vi "Construct.vi"(0 "Components":refnum<class "Component.lvclass">[](array[class]), 11 "error in (no error)":errorcluster) -> (4 "Build Analyzer":refnum<class "Build Analyzer.lvclass">, 15 "error out":errorcluster)   [LabVIEW 2017, in "CL_G3_VIComponentBuilder.lvlib" / "Build Analyzer.lvclass"]
doc: "Generates a hierarchy of components based on an array of \"Component Definition.ini\" files. The set of discovered components is the working set from which build order is determined."
uses:
  Build Analyzer.lvclass
  Components/Component.lvclass
  Exports/Exports/Export.lvclass
  Components/Component.lvclass/Component.ctl
  Build Analyzer.lvclass/Build Analyzer.ctl
  Exports/Exports/Export.lvclass/Export.ctl
  <userlib>/_Cirrus Logic/LabVIEW Container/Source/Container/Container.lvclass/Container.ctl
  Components/Accessors/Read Component Config File.vi
  Components/Accessors/Read Product Name.vi
  Components/Accessors/Read Unique Name.vi
  Accessors/Write Components.vi
  Accessors/Write Component Product Name -_ Unique Name.vi
  <userlib>/_Cirrus Logic/LabVIEW Container/Source/Container/Set N Attributes.vi
  Exports/Exports/Accessors/Read unique Name.vi
  Exports/Exports/Accessors/Read Product Name.vi
  Exports/Exports/Accessors/Read Export Build Specification.vi
  Exports/Exports/Accessors/Read Dependencies' Unique Names.vi
  Exports/Exports/Accessors/Read Owning Component's Product Name.vi
  Exports/Exports/Accessors/Read Owning Component's Unique Name.vi
  Accessors/Write Top Down Working Set.vi
  Accessors/Write Bubble Up Working Set.vi
  <userlib>/_Cirrus Logic/LabVIEW Container/Source/Container/SubVIs/SetAttribute_ByValue.vi
  <userlib>/_Cirrus Logic/LabVIEW Container/Source/Container/Get Child.vi
  <userlib>/_Cirrus Logic/LabVIEW Container/Source/Container/GetAttribute_Path.vi
  <userlib>/_Cirrus Logic/LabVIEW Container/Source/CIR/Interface Definition/Container Intermediate Representation.lvclass
  <userlib>/_Cirrus Logic/LabVIEW Container/Source/Container/Container.lvclass
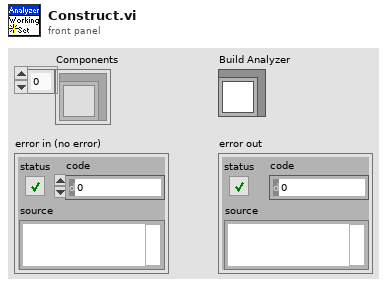
[diagram p1: front panel]
types:
  T1 = cluster{"Build Analyzer":refnum<class "Build Analyzer.lvclass">, "Components":refnum<class "Component.lvclass">[], "Exports":refnum<class "Export.lvclass">[]}
  T2 = enum16{"Overwrite Conflicts", "Error on Conflicts"}
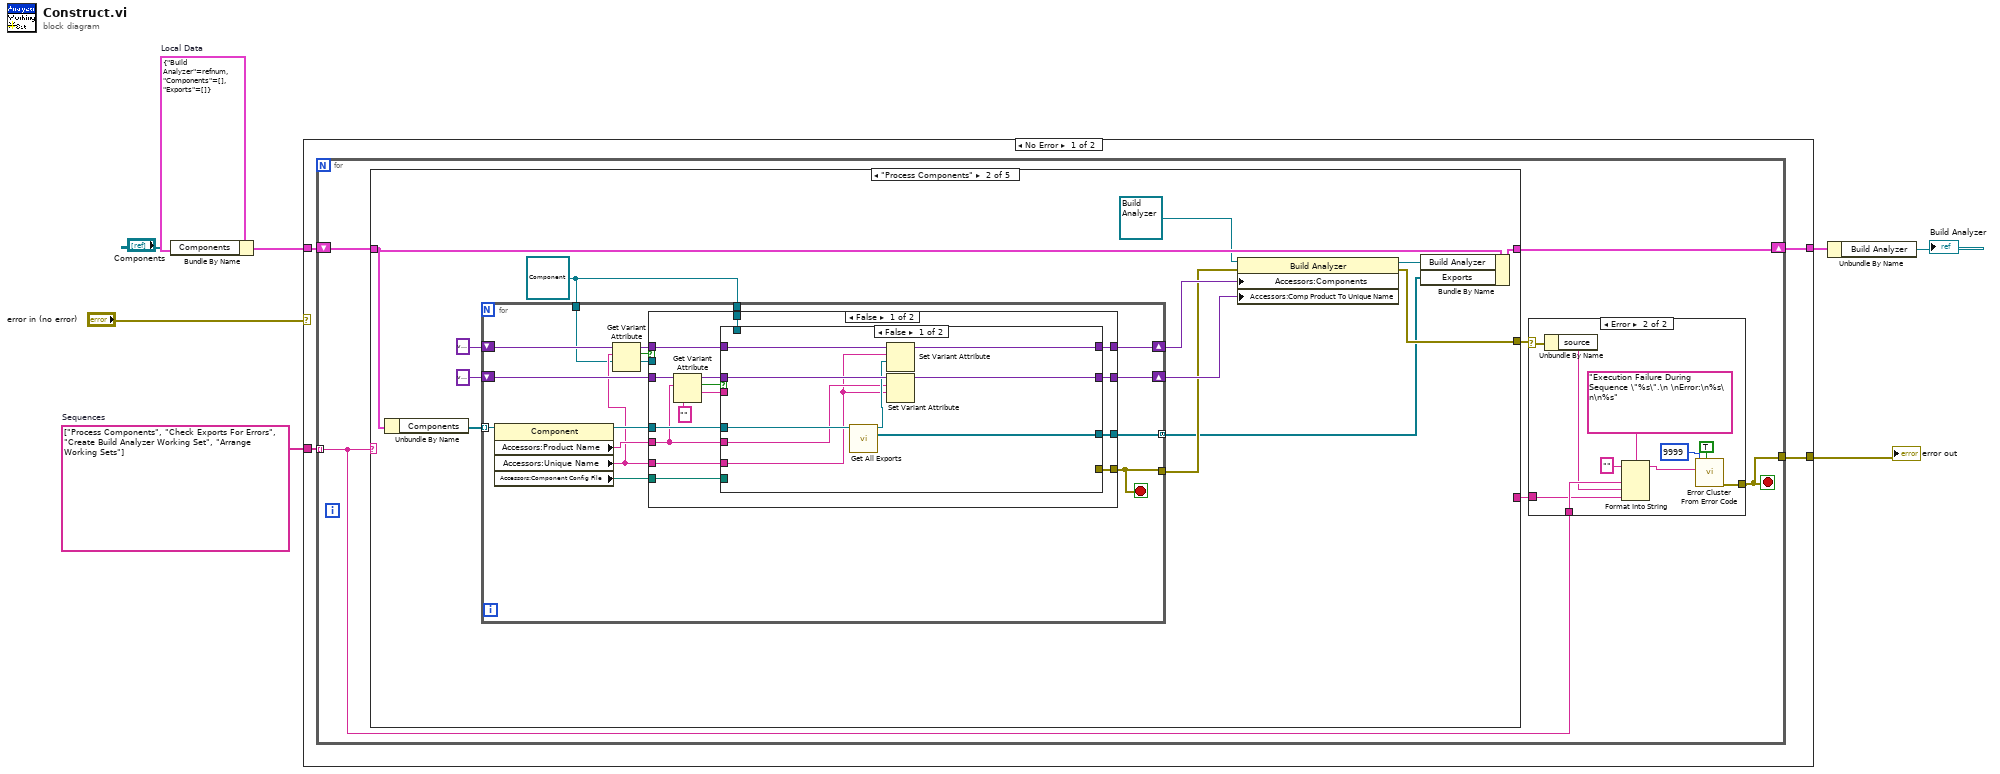
[diagram p0: block diagram]
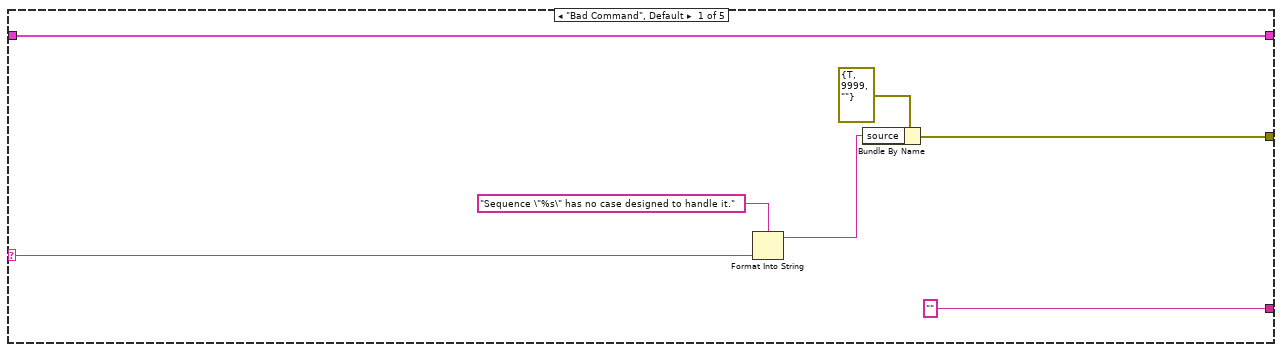
[diagram p3: hidden frame]
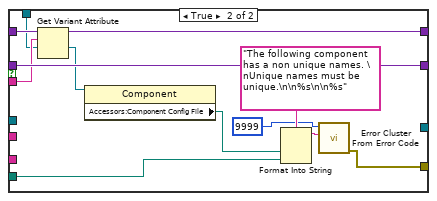
[diagram p4: hidden frame]
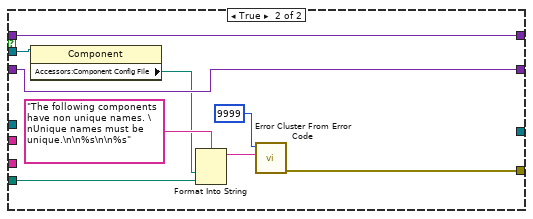
[diagram p5: hidden frame]
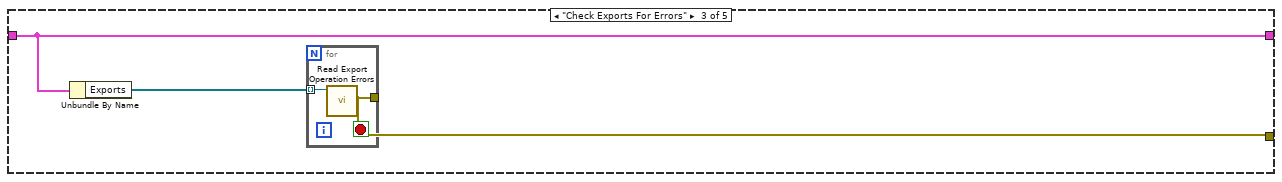
[diagram p6: hidden frame]
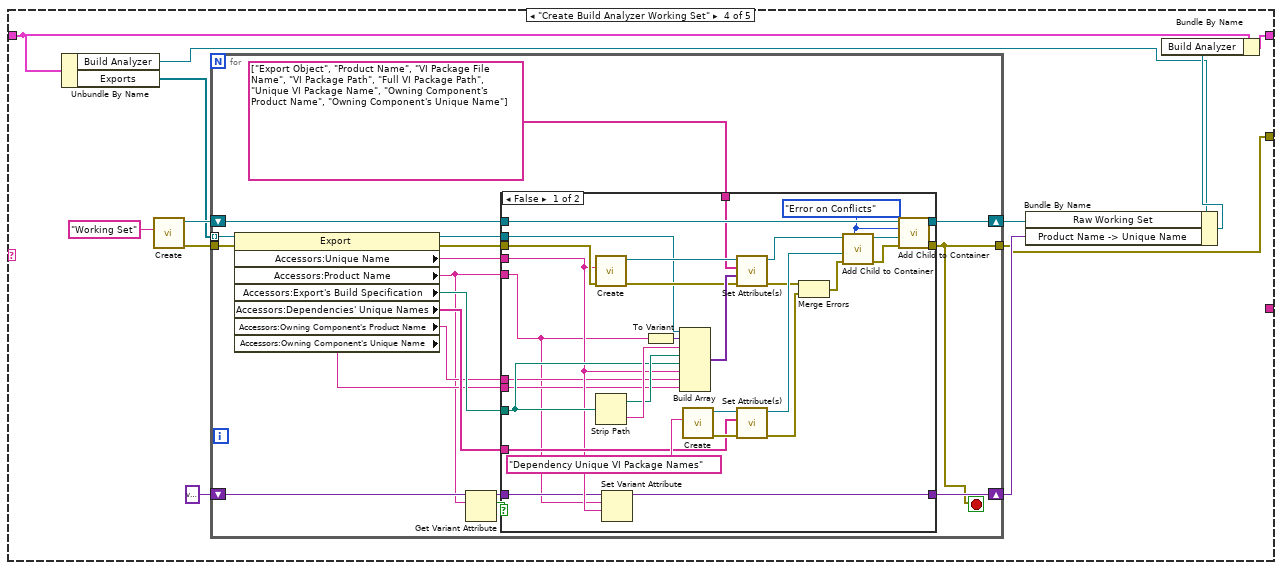
[diagram p7: hidden frame]
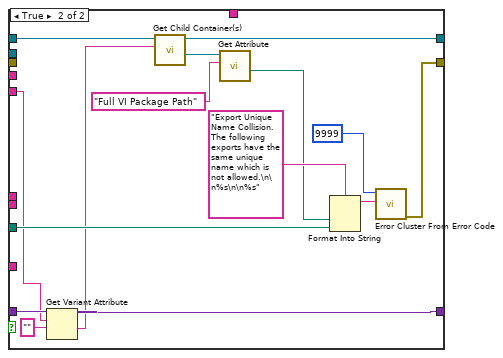
[diagram p8: hidden frame]
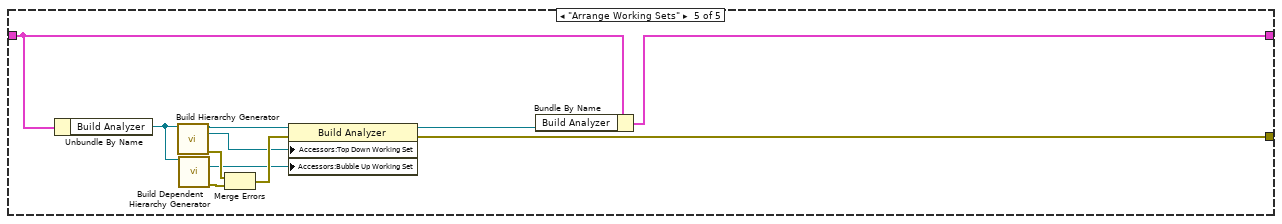
[diagram p9: hidden frame]
diagram:
  w5 = T1 {"Build Analyzer"=refnum, "Components"=[], "Exports"=[]}  # Local Data
  w7 = string[] ["Process Components", "Check Exports For Errors", "Create Build Analyzer Working Set", "Arrange Working Sets"]  # Sequences
  n1 = Bundle By Name(cluster=w5, "Components"="Components") -> (w8:T1)
  n2 = case shown="No Error" "error in (no error)" {
    selector: "error in (no error)" -> [_ w203]
    tunnel: w7 -> [w12 _]
    tunnel: w8 -> [w11 w204]
    tunnel: [w10 w204] -> w6
    tunnel: [w9 w203] -> w2
    frame No Error {
      n3 = for {
        tunnel: w12 -> [w15] mode=indexing
        shift-right: [w17] -> w10
        shift-left: w11 -> [w18]
        tunnel: [w13] -> w9
        stop <- w13 stop-if-true
        n4 = case shown="\"Process Components\"" w15 {
          selector: w15 -> [w31 _ _ _ _]
          tunnel: w18 -> [w36 w47 w113 w123 w202]
          tunnel: [w36 w44 w113 w122 w195] -> w17
          tunnel: [w33 w38 w112 w118 w193] -> w16
          tunnel: ["" ("Accessors:Name") _ _ _ _] -> w14
          frame "Bad Command", Default {
            n5 = Format Into String(format string="Sequence \"%s\" has no case designed to handle it.", w31) -> (resulting string=w30:string)  [unwired: 2 in, 1 out]
            n6 = Bundle By Name(cluster=errorcluster {"status"=TRUE, "code"=9999, "source"=""} ("error out"), "source"=w30) -> (w33:errorcluster)
          }
          frame "Process Components" {
            w43 = refnum<class "Component.lvclass"> refnum ("reference out")
            n7 = Unbundle By Name(w47) -> ("Components"=w46:refnum<class "Component.lvclass">[])
            n8 = for {
              tunnel: [w65] -> w37 mode=concatenating
              shift-right: [w64] -> w41
              shift-left: variant -> [w60]
              shift-right: [w63] -> w42
              shift-left: variant -> [w59]
              tunnel: w46 -> [w61] mode=indexing
              tunnel: [w54] -> w39
              tunnel: w43 -> [w51]
              tunnel: w43 -> [w50]
              stop <- w54 stop-if-true
              n9 = property class="Component"(reference=w61) -> (reference out=w62:refnum<class "Component.lvclass">, "Accessors:Product Name"=w53:string, "Accessors:Unique Name"=w52:string, "Accessors:Component Config File"=w55:path)  [unwired: 1 in, 1 out]
              n10 = Get Variant Attribute(Variant=w59, name=w52, default value (empty Variant)=w51) -> (duplicate Variant=w58:variant, found=w57:bool, value=w56:refnum<class "Component.lvclass">)  [unwired: 1 in, 1 out]
              n11 = case shown="False" w57 {
                tunnel: [w80 _] -> w65
                tunnel: [w79 w108] -> w64
                tunnel: [w78 w109] -> w63
                tunnel: w62 -> [w77 _]
                tunnel: w60 -> [w76 w108]
                tunnel: w58 -> [w70 w109]
                tunnel: w53 -> [w67 _]
                tunnel: w52 -> [w71 _]
                tunnel: w56 -> [_ w110]
                tunnel: w55 -> [w72 w105]
                tunnel: [w73 w103] -> w54
                tunnel: w50 -> [w66 _]
                frame False {
                  n12 = Get Variant Attribute(Variant=w76, name=w67, default value (empty Variant)="") -> (duplicate Variant=w75:variant, found=w74:bool, value=w68:string)  [unwired: 1 in, 1 out]
                  n13 = case shown="False" w74 {
                    tunnel: [w89 _] -> w80
                    tunnel: [w88 w101] -> w79
                    tunnel: [w87 w94] -> w78
                    tunnel: w77 -> [w86 _]
                    tunnel: w75 -> [w85 w101]
                    tunnel: w70 -> [w83 w96]
                    tunnel: w67 -> [w82 _]
                    tunnel: w71 -> [w81 _]
                    tunnel: [_ w98] -> w73
                    tunnel: w72 -> [_ w97]
                    tunnel: w68 -> [_ w95]
                    tunnel: w66 -> [_ w90]
                    frame False {
                      n14 = call "Get All Exports.vi"("Component in"=w86) -> ("Component out"=w84:refnum<class "Component.lvclass">, "Exports"=w89:refnum<class "Export.lvclass">[])  [unwired: 13 in]
                      n15 = Set Variant Attribute(Variant=w83, name=w81, value=w84) -> (Variant out=w87:variant)  [unwired: 1 in, 2 out]
                      n16 = Set Variant Attribute(Variant=w85, name=w82, value=w81) -> (Variant out=w88:variant)  [unwired: 1 in, 2 out]
                    }
                    frame True {
                      n17 = Get Variant Attribute(Variant=w96, name=w95, default value (empty Variant)=w90) -> (duplicate Variant=w94:variant, value=w93:refnum<class "Component.lvclass">)  [unwired: 1 in, 2 out]
                      n18 = property class="Component"(reference=w93) -> ("Accessors:Component Config File"=w92:path)  [unwired: 1 in, 2 out]
                      n19 = Format Into String(format string="The following component has a non unique names. \nUnique names must be unique.\n\n%s\n\n%s", w92, w97) -> (resulting string=w100:string)  [unwired: 2 in, 1 out]
                      n20 = call <vilib>:"Error Cluster From Error Code.vi"("error message (\"\")"=w100, "error code (0)"=9999) -> ("error out"=w98:errorcluster)  [unwired: 7 in]
                    }
                  }
                }
                frame True {
                  n21 = property class="Component"(reference=w110) -> ("Accessors:Component Config File"=w106:path)  [unwired: 1 in, 2 out]
                  n22 = Format Into String(format string="The following components have non unique names. \nUnique names must be unique.\n\n%s\n\n%s", w106, w105) -> (resulting string=w104:string)  [unwired: 2 in, 1 out]
                  n23 = call <vilib>:"Error Cluster From Error Code.vi"("error message (\"\")"=w104, "error code (0)"=9999) -> ("error out"=w103:errorcluster)  [unwired: 7 in]
                }
              }
            }
            n24 = property class="Build Analyzer"(reference=refnum<class "Build Analyzer.lvclass"> refnum ("Build Analyzer.lvclass"), error in=w39, "Accessors:Components"=w42, "Accessors:Comp Product To Unique Name"=w41) -> (reference out=w40:refnum<class "Build Analyzer.lvclass">, error out=w38:errorcluster)
            n25 = Bundle By Name(cluster=w47, "Build Analyzer"=w40, "Exports"=w37) -> (w44:T1)
          }
          frame "Check Exports For Errors" {
            n26 = Unbundle By Name(w113) -> ("Exports"=w111:refnum<class "Export.lvclass">[])
            n27 = for {
              tunnel: w111 -> [w115] mode=indexing
              tunnel: [w114] -> w112
              stop <- w114 stop-if-true
              n28 = call "Read Export Operation Errors.vi"("Export in"=w115) -> ("Export Operation Errors"=w114:errorcluster)  [unwired: 8 in, 2 out]
            }
          }
          frame "Create Build Analyzer Working Set" {
            n29 = Unbundle By Name(w123) -> ("Build Analyzer"=w117:refnum<class "Build Analyzer.lvclass">, "Exports"=w116:refnum<class "Export.lvclass">[])
            n30 = call <userlib>:"Create.vi"("Container Name"="Working Set") -> ("error out"=w125:errorcluster, "Container"=w127:refnum<data-value>)  [unwired: 9 in]
            n31 = for {
              shift-right: [w143] -> w120
              shift-left: w127 -> [w145]
              tunnel: w116 -> [w137] mode=indexing
              shift-right: [w138] -> w119
              shift-left: variant -> [w133]
              tunnel: w125 -> [w136]
              tunnel: [w131] -> w118
              stop <- w131 stop-if-true
              n32 = property class="Export"(reference=w137, error in=w136) -> (reference out=w140:refnum<class "Export.lvclass">, error out=w141:errorcluster, "Accessors:Unique Name"=w129:string, "Accessors:Product Name"=w128:string, "Accessors:Export's Build Specification"=w142:path, "Accessors:Dependencies' Unique Names"=w139:string[], "Accessors:Owning Component's Product Name"=w135:string, "Accessors:Owning Component's Unique Name"=w134:string)
              n33 = Get Variant Attribute(Variant=w133, name=w128) -> (duplicate Variant=w132:variant, found=w130:bool)  [unwired: 2 in, 2 out]
              n34 = case shown="False" w130 {
                tunnel: w145 -> [w176 w184]
                tunnel: string[] ["Export Object", "Product Name", "VI Package File Name", "VI Package Path", "Full VI Package Path", "Unique VI Package Name", "Owning Component's Product Name", "Owning Component's Unique Name"] ("Attribute Names") -> [w174 _]
                tunnel: [w169 w182] -> w143
                tunnel: w142 -> [w163 w189]
                tunnel: w141 -> [w162 _]
                tunnel: w140 -> [w155 _]
                tunnel: w139 -> [w154 _]
                tunnel: [w153 w177] -> w138
                tunnel: w129 -> [w152 _]
                tunnel: w135 -> [w151 _]
                tunnel: w134 -> [w150 _]
                tunnel: w132 -> [w149 w181]
                tunnel: w128 -> [w148 w180]
                tunnel: [w147 w186] -> w131
                frame False {
                  w146 = T2."Error on Conflicts" ("Overwrite behavior")
                  n35 = call <userlib>:"Create.vi"("error in (no error)"=w162, "Container Name"=w152) -> ("error out"=w161:errorcluster, "Container"=w175:refnum<data-value>)  [unwired: 8 in]
                  n36 = Strip Path(path=w163) -> (stripped path=w172:path, name=w173:string)
                  n37 = Set Variant Attribute(Variant=w149, name=w148, value=w152) -> (Variant out=w153:variant)  [unwired: 1 in, 2 out]
                  n38 = To Variant(anything=w148) -> (Variant=w170:variant)
                  n39 = Build Array(w155, w170, w173, w172, w163, w152, w151, w150) -> (w171:variant[])
                  n40 = call <userlib>:"Create.vi"("Container Name"="Dependency Unique VI Package Names") -> ("error out"=w160:errorcluster, "Container"=w165:refnum<data-value>)  [unwired: 9 in]
                  n41 = call-poly <userlib>:"Set Attribute(s).vi"("error in"=w161, "Attribute Values"=w171, "Attribute Names"=w174, "Container"=w175) -> ("error out"=w159:errorcluster, "Container out"=w167:refnum<data-value>)  [unwired: 5 in, 1 out]
                  n42 = call-poly <userlib>:"Set Attribute(s).vi"("error in"=w160, "Attribute Names"=w154, "Container"=w165) -> ("error out"=w158:errorcluster, "Container out"=w164:refnum<data-value>)  [unwired: 6 in, 1 out]
                  n43 = Merge Errors(w159, w158) -> (w157:errorcluster)
                  n44 = call <userlib>:"Add Child to Container.vi"("Overwrite behavior"=w146, "error in (no error)"=w157, "Child Container"=w164, "Container"=w167) -> ("error out"=w156:errorcluster, "dup Container"=w166:refnum<data-value>)  [unwired: 5 in, 1 out]
                  n45 = call <userlib>:"Add Child to Container.vi"("Overwrite behavior"=w146, "error in (no error)"=w156, "Child Container"=w166, "Container"=w176) -> ("error out"=w147:errorcluster, "dup Container"=w169:refnum<data-value>)  [unwired: 5 in, 1 out]
                }
                frame True {
                  n46 = Get Variant Attribute(Variant=w181, name=w180, default value (empty Variant)="") -> (duplicate Variant=w177:variant, value=w178:string)  [unwired: 1 in, 2 out]
                  n47 = call-poly <userlib>:"Get Child Container(s).vi"("Container Name"=w178, "Container"=w184) -> ("Child Container"=w183:refnum<data-value>, "dup Container"=w182:refnum<data-value>)  [unwired: 6 in, 2 out]
                  n48 = call-poly <userlib>:"Get Attribute.vi"("Attribute Name"="Full VI Package Path", "Container Reference"=w183) -> ("Path"=w188:path)  [unwired: 6 in, 3 out]
                  n49 = Format Into String(format string="Export Unique Name Collision. The following exports have the same unique name which is not allowed.\n\n%s\n\n%s", w188, w189) -> (resulting string=w187:string)  [unwired: 2 in, 1 out]
                  n50 = call <vilib>:"Error Cluster From Error Code.vi"("error message (\"\")"=w187, "error code (0)"=9999) -> ("error out"=w186:errorcluster)  [unwired: 7 in]
                }
              }
            }
            n51 = Bundle By Name(cluster=w117, "Raw Working Set"=w120, "Product Name -> Unique Name"=w119) -> (w121:refnum<class "Build Analyzer.lvclass">)
            n52 = Bundle By Name(cluster=w123, "Build Analyzer"=w121) -> (w122:T1)
          }
          frame "Arrange Working Sets" {
            n53 = Unbundle By Name(w202) -> ("Build Analyzer"=w196:refnum<class "Build Analyzer.lvclass">)
            n54 = call "Build Hierarchy Generator.vi"("Build Analyzer in"=w196) -> ("dup Build Analyzer"=w192:refnum<class "Build Analyzer.lvclass">, "Top Down Working Set"=w197:refnum<data-value>, "error out"=w201:errorcluster)  [unwired: 12 in]
            n55 = call "Build Dependent Hierarchy Generator.vi"("Build Analyzer in"=w196) -> ("Bubbe Up Working Set"=w198:refnum<data-value>, "error out"=w200:errorcluster)  [unwired: 12 in, 1 out]
            n56 = Merge Errors(w201, w200) -> (w199:errorcluster)
            n57 = property class="Build Analyzer"(reference=w192, error in=w199, "Accessors:Top Down Working Set"=w197, "Accessors:Bubble Up Working Set"=w198) -> (reference out=w194:refnum<class "Build Analyzer.lvclass">, error out=w193:errorcluster)
            n58 = Bundle By Name(cluster=w202, "Build Analyzer"=w194) -> (w195:T1)
          }
        }
        n59 = case shown="Error" w16 {
          selector: w16 -> [w19 w22]
          tunnel: [w19 w27] -> w13
          tunnel: w15 -> [_ w25]
          tunnel: w14 -> [_ w20]
          frame No Error {
          }
          frame Error {
            n60 = Unbundle By Name(w22) -> ("source"=w21:string)
            n61 = Format Into String(format string="Execution Failure During Sequence \"%s\".\n \nError:\n%s\n\n%s" ("error message (\"\")"), initial string="", w25, w21, w20) -> (resulting string=w26:string)  [unwired: 1 in, 1 out]
            n62 = call <vilib>:"Error Cluster From Error Code.vi"("show call chain? (False)"=TRUE, "error message (\"\")"=w26, "error code (0)"=9999) -> ("error out"=w27:errorcluster)  [unwired: 6 in]
          }
        }
      }
    }
    frame Error {
    }
  }
  "error out" <- w2
  n63 = Unbundle By Name(w6) -> ("Build Analyzer"=→"Build Analyzer":refnum<class "Build Analyzer.lvclass">)
